vi "_CommonPage.vi"(11 "DB Ref":T1) -> (2 "Value String":string, 3 "Boolean":bool)   [LabVIEW 2017]
uses:
  Typedef/TagDB.ctl
  DataAccess/_NameCacher.vi
  DataAccess/TagDB Ref to DVR.vi
  Error/_[error50000]Invalid DB REF.vi
  <vilib>/Utility/error.llb/Trim Whitespace.vi
  TagDB(DEV).lvlib
panel:
  out "Valid?":bool
  out "Name":string
  out "DataItemFlag":timestamp
  out "DataChangeFlag":timestamp
  in  "Items":i32(listbox)
  out "VI Server Type":T2(ring)
  out "Data Type":T3(ring)
  out "data":variant
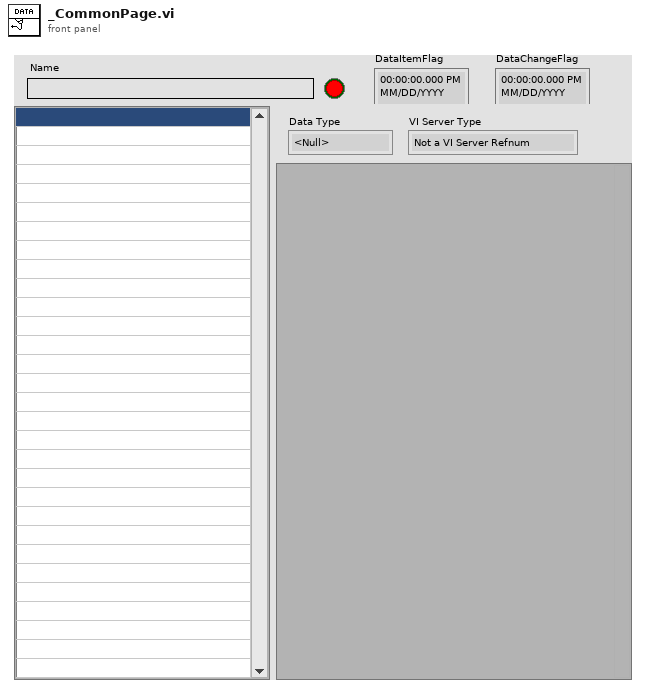
[diagram p1: front panel]
types:
  T1 = typedef "TagDB(DEV).lvlib/TagDB.ctl" = refnum<k1>
  T2 = enum16{"Not a VI Server Refnum", "Control", "VI", "Application", "Splitter", "Pane"}
  T3 = enum8{"<Null>", "I8", "I16", "I32", "I64", "U8", "U16", "U32", "U64", "SGL", "DBL", "EXT", "CSG", "CDB", "CXT", "0x0F", "0x10", "0x11", "0x12", "0x13", "0x14", "Enum U8", "Enum U16", "Enum U32", "Enum U64", "SGL PQ", "DBL PQ", "EXT PQ", "CSG PQ", "CDB PQ", "CXT PQ", "0x1F", "0x20", "Boolean", "0x22", "0x23", "0x24", "0x25", "0x26", "0x27", "0x28", "0x29", "0x2A", "0x2B", "0x2C", "0x2D", "0x2E", "0x2F", "String", "0x31", "Path", "Pict", "0x34", "0x35", "0x36", "DAQ", "0x38", "0x39", "0x3A", "0x3B", "0x3C", "0x3D", "0x3E", "0x3F", "Array", "0x41", "0x42", "0x43", "0x44", "0x45", "0x46", "0x47", "0x48", "0x49", "0x4A", "0x4B", "0x4C", "0x4D", "0x4E", "0x4F", "Cluster", "0x51", "0x52", "Variant", "Waveform", "0x55", "0x56", "0x57", "0x58", "0x59", "0x5A", "0x5B", "0x5C", "0x5D", "0x5E", "0x5F", "0x60", "0x61", "0x62", "0x63", "0x64", "0x65", "0x66", "0x67", "0x68", "0x69", "0x6A", "0x6B", "0x6C", "0x6D", "0x6E", "0x6F", "Refnum"}
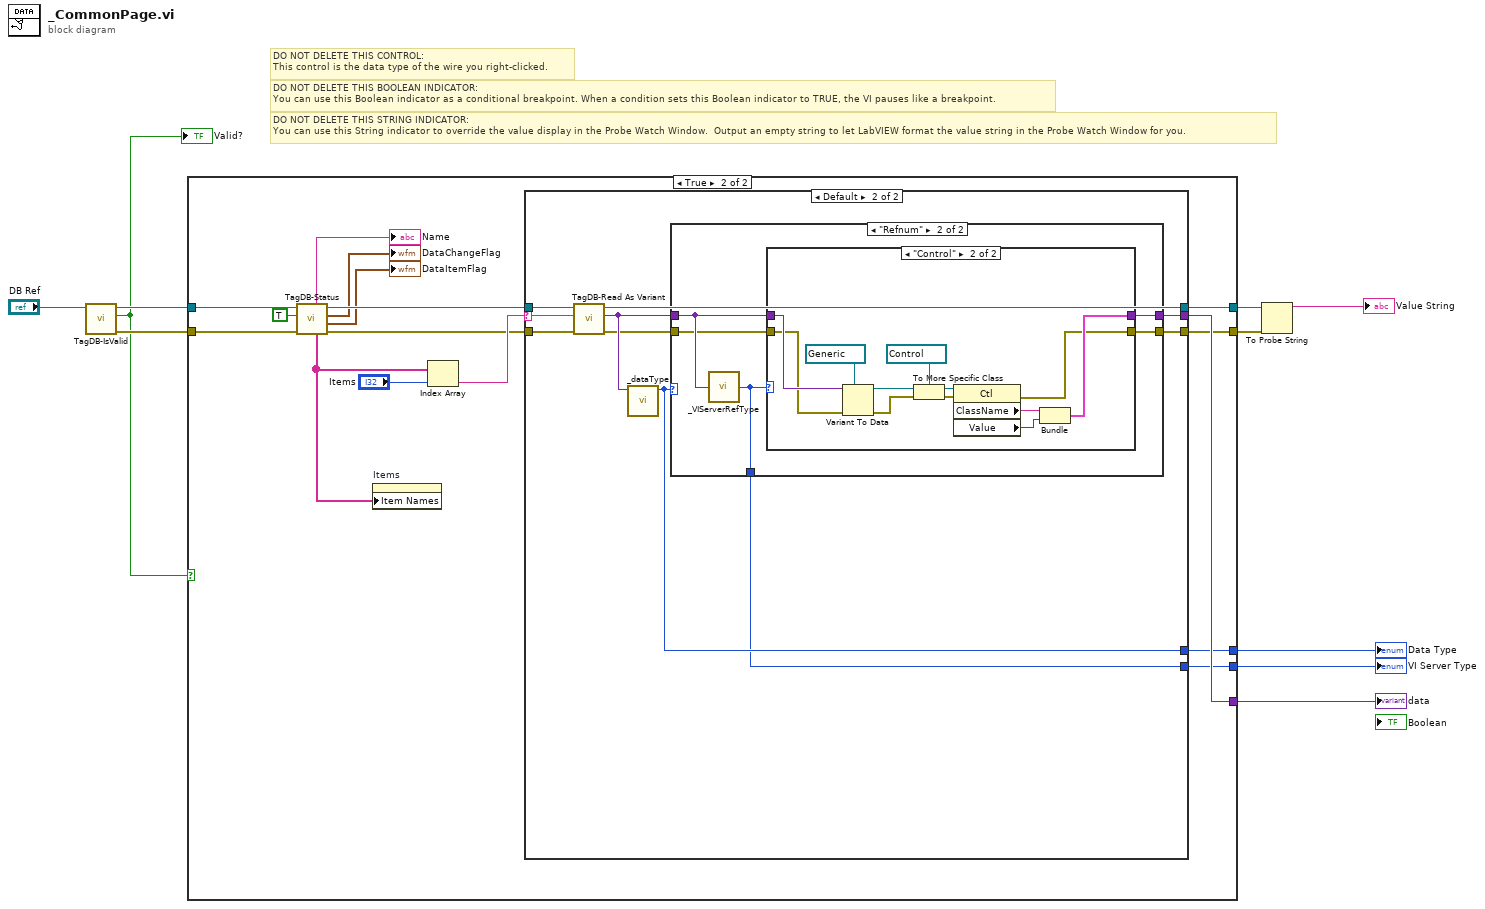
[diagram p0: block diagram]
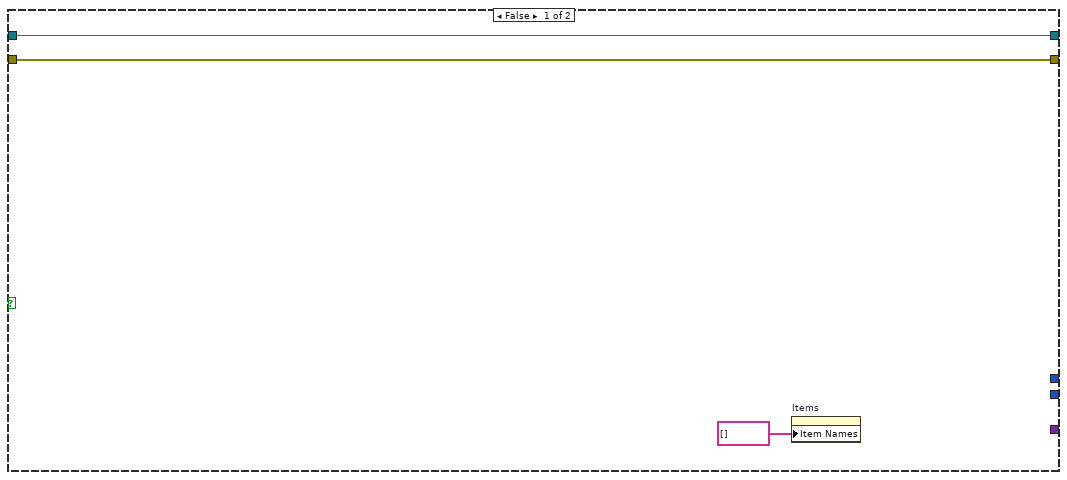
[diagram p2: hidden frame]
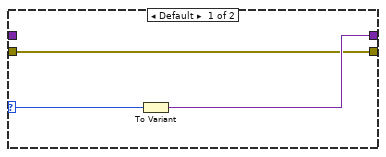
[diagram p5: hidden frame]
diagram:
  # "DO NOT DELETE THIS STRING INDICATOR: \nYou can use this String indicator to override the value display in the Probe Watch Window.  Output an empty string to let LabVIEW format the value string in the Probe Watch Window for you."
  # "DO NOT DELETE THIS BOOLEAN INDICATOR: \nYou can use this Boolean indicator as a conditional breakpoint. When a condition sets this Boolean indicator to TRUE, the VI pauses like a breakpoint."
  # "DO NOT DELETE THIS CONTROL: \nThis control is the data type of the wire you right-clicked."
  n1 = call <userlib>:"TagDB-IsValid.vi"("TagDB"="DB Ref") -> ("error out"=w6:errorcluster, "valid TagDB?"=w3:bool, "TagDB(dup)"=w7:T1)  [unwired: 8 in]
  "Valid?" <- w3
  n2 = case shown="True" w3 {
    tunnel: [_ w29] -> w8
    tunnel: w7 -> [w13 w28]
    tunnel: w6 -> [w12 w20]
    tunnel: [w13 w27] -> w5
    tunnel: [w12 w26] -> w4
    tunnel: [_ w23] -> w2
    tunnel: [_ w22] -> w1
    frame False {
      n3 = property on="Items" class="LstBox (strict)"("Item Names"=string[] []) -> ()  [unwired: 2 in, 2 out]
    }
    frame True {
      n4 = call "TagDB-Status.vi"("error in (no error)"=w20, "return elements? (F)"=TRUE, "DB Ref"=w28) -> ("error out"=w15:errorcluster, "Item Change Timestamp"=→"DataItemFlag":timestamp, "Global Change Timestamp"=→"DataChangeFlag":timestamp, "DB Ref(dup)"=w21:T1, "DB items"=w14:string[], "db name"=→"Name":string)  [unwired: 3 in]
      n5 = property on="Items" class="LstBox (strict)"("Item Names"=w14) -> ()  [unwired: 2 in, 2 out]
      n6 = Index Array(array=w14, index="Items") -> (element=w24:string)
      n7 = case shown="Default" w24 {
        selector: w24 -> [_ w40]
        tunnel: w21 -> [w31 w41]
        tunnel: [w31 w39] -> w27
        tunnel: [w30 w34] -> w26
        tunnel: [_ w37] -> w29
        tunnel: w15 -> [w30 w38]
        tunnel: [_ w33] -> w23
        tunnel: [_ w32] -> w22
        frame "" {
        }
        frame Default {
          n8 = call "TagDB-Read As Variant.vi"("error in (no error)"=w38, "name"=w40, "TagDB"=w41) -> ("error out"=w35:errorcluster, "Value"=w36:variant, "TagDB(dup)"=w39:T1)  [unwired: 3 in, 3 out]
          n9 = call "_dataType.vi"("Type"=w36) -> ("type"=w33:T3)  [unwired: 10 in]
          n10 = case shown="\"Refnum\"" w33 {
            tunnel: [w43 w48] -> w37
            tunnel: w36 -> [w43 w47]
            tunnel: w35 -> [w42 w46]
            tunnel: [w42 w45] -> w34
            tunnel: [_ w44] -> w32
            frame Default {
            }
            frame "Refnum" {
              n11 = call "_VIServerRefType.vi"("Data"=w47) -> ("Enum"=w44:T2)  [unwired: 4 in]
              n12 = case shown="\"Control\"" w44 {
                selector: w44 -> [w51 _]
                tunnel: [w50 w54] -> w48
                tunnel: w47 -> [_ w63]
                tunnel: w46 -> [w49 w53]
                tunnel: [w49 w52] -> w45
                frame Default {
                  n13 = To Variant(anything=w51) -> (Variant=w50:variant)
                }
                frame "Control" {
                  n14 = Variant To Data(error in=w53, type=refnum<vi> refnum ("value"), Variant=w63) -> (data=w61:refnum<vi>, error out=w60:errorcluster)
                  n15 = To More Specific Class(target class=refnum<vi> refnum ("value"), reference=w61, error in=w60) -> (specific class reference=w58:refnum<vi>, error out=w57:errorcluster)
                  n16 = property class="Ctl"(reference=w58, error in=w57) -> (error out=w52:errorcluster, "ClassName"=w56:string, "Value"=w55:variant)  [unwired: 1 out]
                  n17 = Bundle("ClassName"=w56, "Value"=w55) -> (w54:cluster{"ClassName":string, "Value":variant})  [unwired: 1 in]
                }
              }
            }
          }
        }
      }
    }
  }
  "data" <- w8
  "Data Type" <- w2
  "VI Server Type" <- w1
  n18 = To Probe String(4:w4, 7:w5) -> (3:→"Value String":string)  [unwired: 1 in, 1 out]
